vi "setUp.vi"(8 "error in (no error)":errorcluster, 11 "reference in":refnum<class "FPGA Addon Scalar Channels System Tests.lvclass">) -> (0 "error out":errorcluster, 3 "reference out":refnum<class "FPGA Addon Scalar Channels System Tests.lvclass">)   [LabVIEW 2018, in "FPGA Addon Scalar Channels System Tests.lvclass"]
doc: "setUp runs prior to the test method during test execution. Use this method to initialize any object data required by your tests."
uses:
  FPGA Addon Scalar Channels System Tests.lvclass
  C:/Users/nitest/Desktop/NI VS FPGA Addon CD Fork/Source/Tests/FPGA Addon Test Class/FPGA Addon Test Class.lvclass
  FPGA Addon Test Class/FPGA Addon Test Class.lvclass/FPGA Addon Test Class.ctl
  FPGA Addon Test Class/FPGA Addon Test Class.lvclass
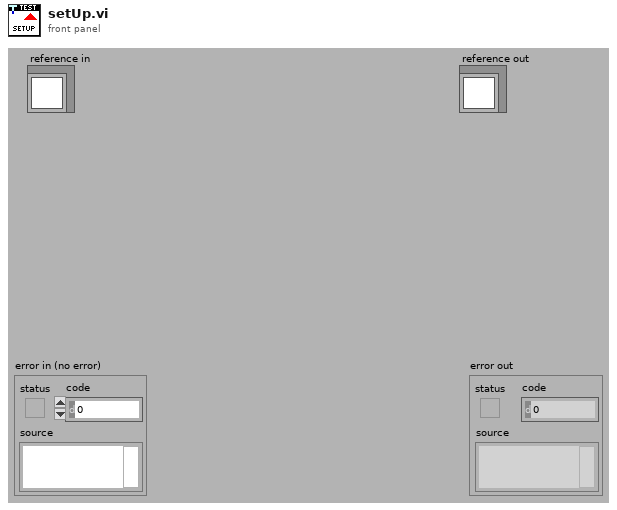
[diagram p1: front panel]
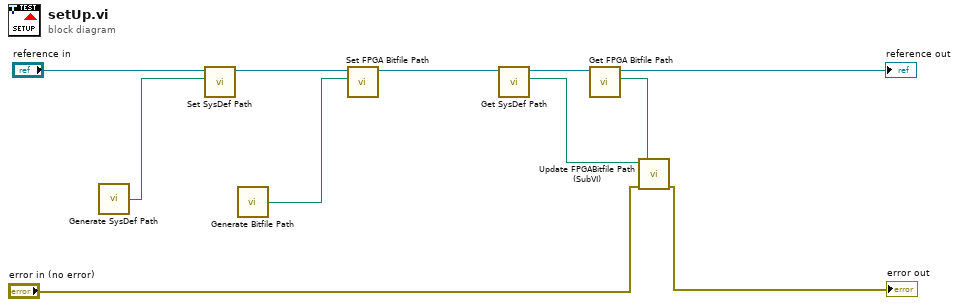
[diagram p0: block diagram]
diagram:
  n1 = call "Generate SysDef Path.vi"() -> ("System Definition path"=w8:path)
  n2 = call "Set SysDef Path.vi"("SysDef Path"=w8, "Scalar Channels Testing in"="reference in") -> ("Scalar Channels Testing out"=w7:refnum<class "FPGA Addon Scalar Channels System Tests.lvclass">)  [unwired: 9 in]
  n3 = call "Generate Bitfile Path.vi"() -> ("Bitfile Path"=w6:path)
  n4 = call "Set FPGA Bitfile Path.vi"("FPGA Bitfile Path"=w6, "Scalar Channels Testing in"=w7) -> ("Scalar Channels Testing out"=w5:refnum<class "FPGA Addon Scalar Channels System Tests.lvclass">)  [unwired: 9 in]
  n5 = call "Get SysDef Path.vi"("Scalar Channels Testing in"=w5) -> ("SysDef Path"=w1:path, "Scalar Channels Testing out"=w4:refnum<class "FPGA Addon Scalar Channels System Tests.lvclass">)  [unwired: 9 in]
  n6 = call "Get FPGA Bitfile Path.vi"("Scalar Channels Testing in"=w4) -> ("FPGA Bitfile Path"=w2:path, "Scalar Channels Testing out"=→"reference out":refnum<class "FPGA Addon Scalar Channels System Tests.lvclass">)  [unwired: 9 in]
  n7 = call "Update FPGABitfile Path (SubVI).vi"("Bitfile Path"=w2, "error in (no error)"="error in (no error)", "System Definition path in"=w1) -> ("error out"=→"error out":errorcluster)  [unwired: 7 in, 1 out]
